vi "Pre Launch Init.vi"(11 "Nested in":refnum<class "ATM_UI_Controller.lvclass">) -> (0 "error out":errorcluster, 3 "Nested out":refnum<class "ATM_UI_Controller.lvclass">)   [LabVIEW 2025, in "ATM_UI_Controller.lvlib" / "ATM_UI_Controller.lvclass"]
doc: "(<B>Filename</B>: Actor Framework.lvlib:Actor.lvclass:Pre Launch Init.vi)\n\nDefines behavior that occurs after the Launch Nested Actor method is invoked but before the actor's Actor Core method begins running.\n\nBy default, this method does nothing. A descendant class may override it to define behavior."
uses:
  ATM_UI_Controller.lvclass
  ATM_UI_Controller.lvclass/ATM_UI_Controller.ctl
  <vilib>/ni/Actors/State Actor/State Actor/State Actor.lvclass
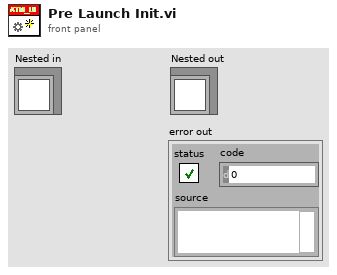
[diagram p1: front panel]
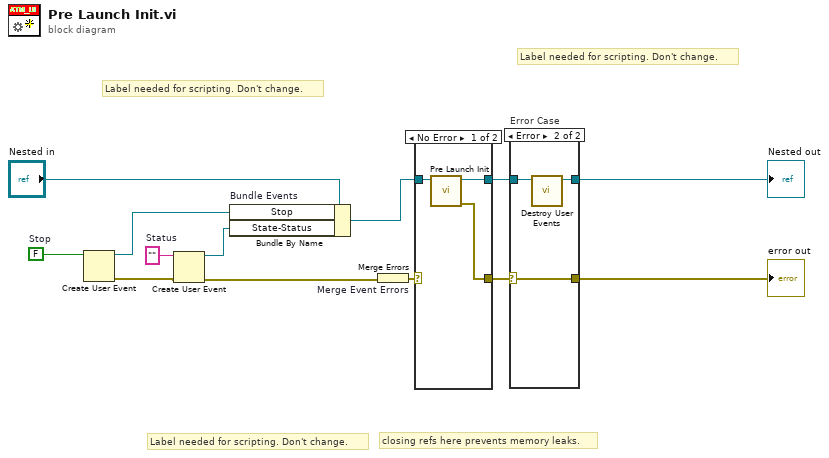
[diagram p0: block diagram]
diagram:
  w1 = ""  # Status
  w5 = FALSE  # Stop
  # "Label needed for scripting. Don't change."
  # "Label needed for scripting. Don't change."
  # "Label needed for scripting. Don't change."
  # "closing refs here prevents memory leaks."
  n1 = Create User Event(user event datatype=w5) -> (user event=w11:refnum<user-event>, error out=w4:errorcluster)  [unwired: 1 in]
  n2 = Create User Event(user event datatype=w1, error in=w4) -> (user event=w2:refnum<user-event>, error out=w3:errorcluster)
  n3 = Bundle By Name "Bundle Events"(cluster="Nested in", "Stop"=w11, "State-Status"=w2) -> (w8:refnum<class "ATM_UI_Controller.lvclass">)
  n4 = Merge Errors "Merge Event Errors"(w3) -> (w7:errorcluster)
  n5 = case shown="No Error" w7 {
    selector: w7 -> [_ w18]
    tunnel: [w16 w17] -> w9
    tunnel: w8 -> [w15 w17]
    tunnel: [w14 w18] -> w6
    frame No Error {
      n6 = call-parent "Pre Launch Init.vi"("Actor in"=w15) -> ("error out"=w14:errorcluster, "Actor out"=w16:refnum<class "ATM_UI_Controller.lvclass">)  [unwired: 9 in]
    }
    frame Error {
    }
  }
  n7 = case "Error Case" shown="Error" w6 {
    selector: w6 -> [w19 w23]
    tunnel: w9 -> [w20 w22]
    tunnel: [w20 w21] -> w12
    tunnel: [w19 w23] -> w10
    frame No Error {
    }
    frame Error {
      n8 = call "Destroy User Events.vi"("UI Template in"=w22) -> ("UI Template out"=w21:refnum<class "ATM_UI_Controller.lvclass">)  [unwired: 10 in]
    }
  }
  "error out" <- w10
  "Nested out" <- w12
